vi "http handle content data.vi"(4 "transmit queue":refnum<queue>, 6 "exec queue":refnum<queue>, 9 "server properties":T1={"max url size"=8000, "max header"=8000, "timeout ms"=5000, "max data size"=104857600}, 10 "application request":T2, 11 "TCP Network Connection in":refnum<k5>) -> (3 "abort":bool)   [LabVIEW 2013, in "Basic HTTP server.lvclass"]
uses:
  Basic HTTP server.lvclass
  http request.ctl
  http method.ctl
  URI/url structure.ctl
  HTTP headers/http header data.ctl
  http response.ctl
  http response packet type.ctl
  http server properties.ctl
  http chunked encoding state.ctl
  <vilib>/dlg_ctls.llb/Space Constant.vi
  HTTP headers/http add header to set.vi
  HTTP headers/http headers.lvlib
  URI/uniform resource locator.lvlib
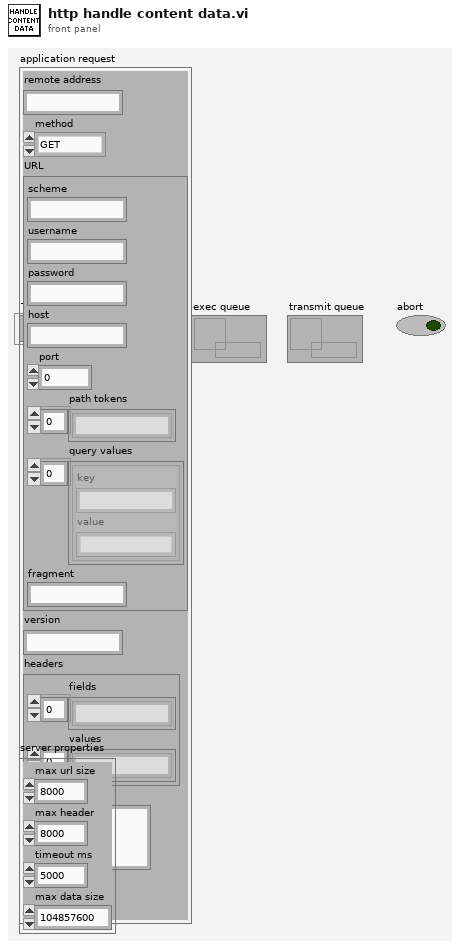
[diagram p1: front panel]
types:
  T1 = typedef "Basic HTTP server.lvclass/http server properties.ctl" = cluster{"max url size":i32, "max header":i32, "timeout ms":i32, "max data size":i32}
  T2 = typedef "Basic HTTP server.lvclass/http request.ctl" = cluster{"remote address":string, "method":T3, "URL":T4, "version":string, "headers":T5, "data":string, "has data?":bool}
  T3 = typedef "Basic HTTP server.lvclass/http method.ctl" = enum16{"GET", "POST", "PUT", "DELETE", "HEAD", "OPTIONS", "upgrade"}
  T4 = typedef "uniform resource locator.lvlib/url structure.ctl" = cluster{"scheme":string, "username":string, "password":string, "host":string, "port":u16, "path tokens":string[], "query values":cluster{"key":string, "value":string}[], "fragment":string}
  T5 = typedef "http headers.lvlib/http header data.ctl" = cluster{"fields":string[], "values":string[]}
  T6 = typedef "Basic HTTP server.lvclass/http chunked encoding state.ctl" = enum16{"length", "data", "trailer"}
  T7 = enum16{"Standard", "Buffered", "CRLF", "Immediate"}
  T8 = typedef "Basic HTTP server.lvclass/http response.ctl" = cluster{"packet type":T9, "reason code":u16, "status string":string, "headers":T5, "cookies":string[], "data":string}
  T9 = typedef "Basic HTTP server.lvclass/http response packet type.ctl" = enum16{"full response", "header only", "data only", "last data"}
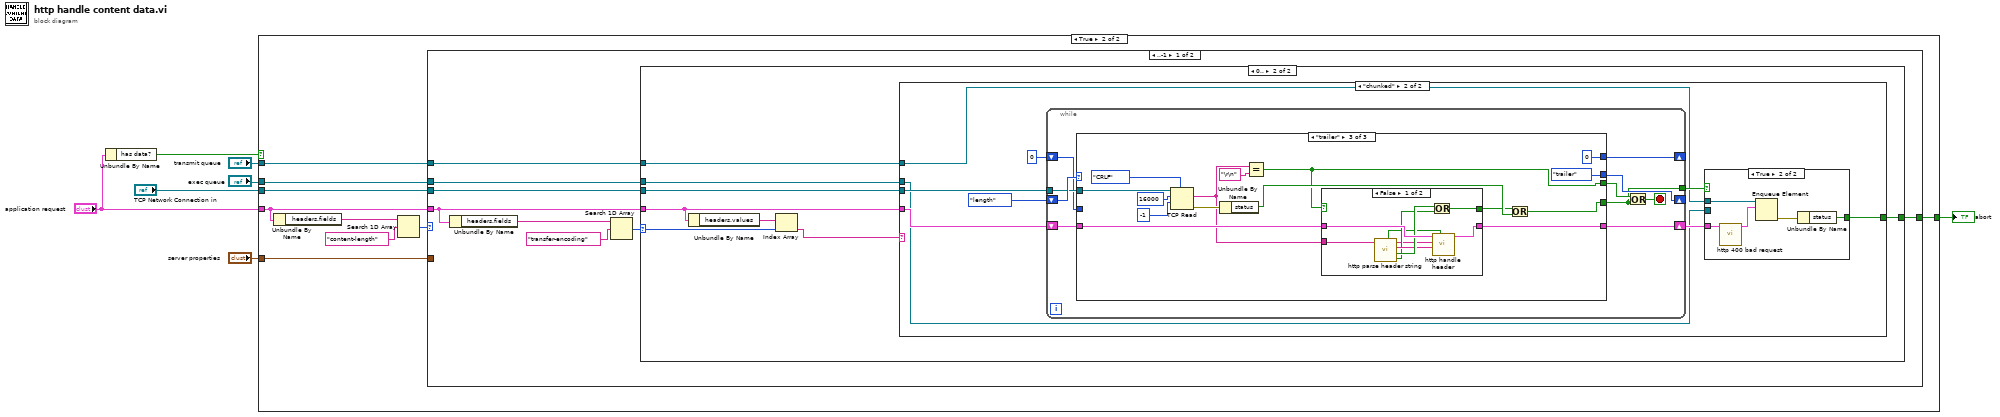
[diagram p0: block diagram]
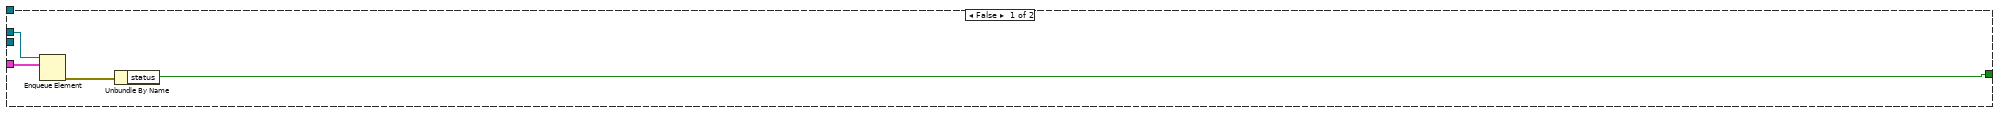
[diagram p2: hidden frame]
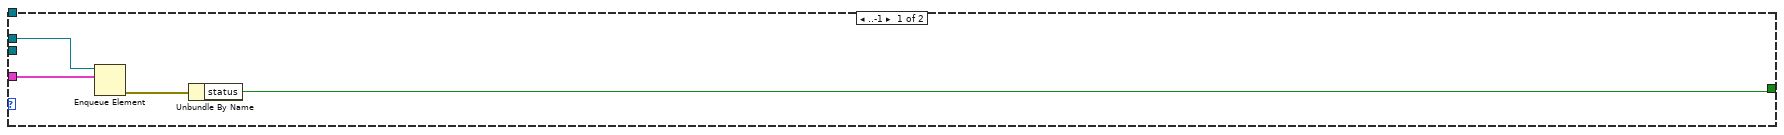
[diagram p3: hidden frame]
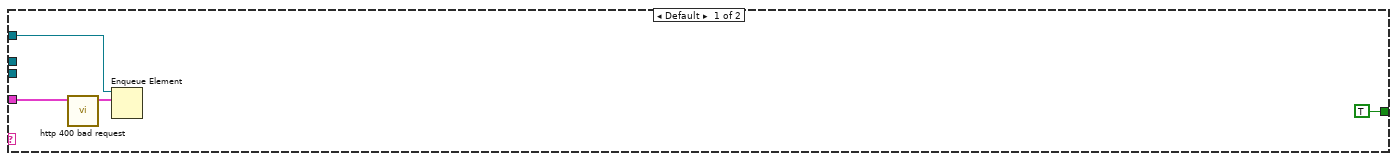
[diagram p4: hidden frame]
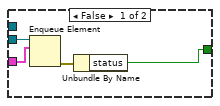
[diagram p5: hidden frame]
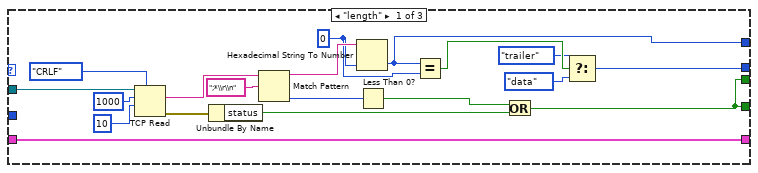
[diagram p6: hidden frame]
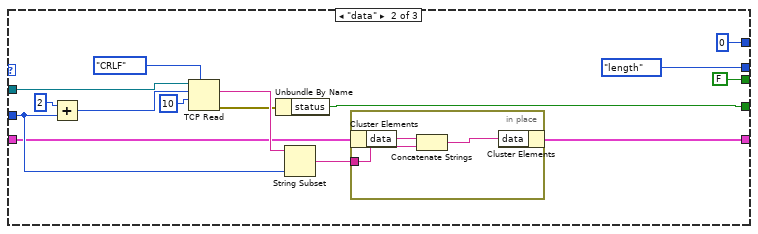
[diagram p7: hidden frame]
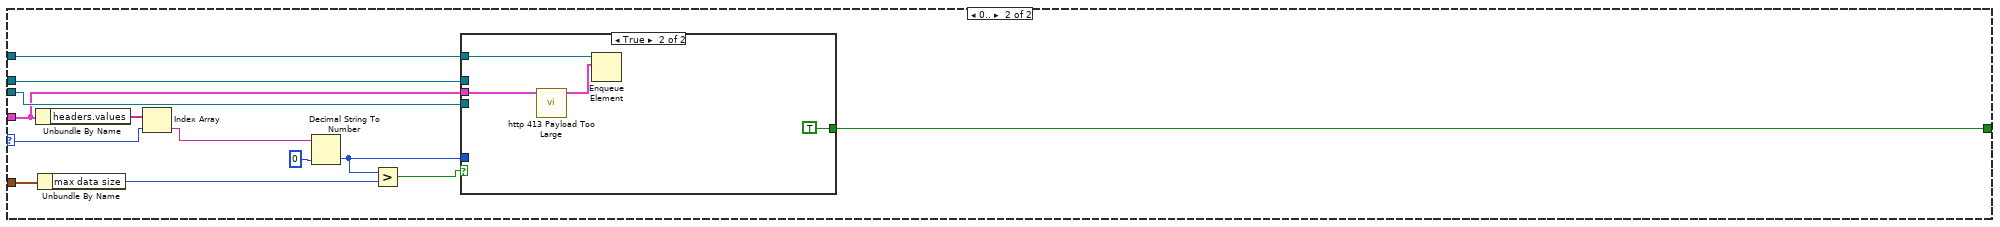
[diagram p9: hidden frame]
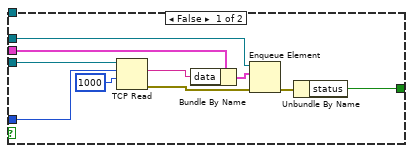
[diagram p10: hidden frame]
diagram:
  n1 = Unbundle By Name("application request") -> ("has data?"=w1:bool)
  n2 = case shown="True" w1 {
    tunnel: "TCP Network Connection in" -> [_ w20]
    tunnel: [w8 w19] -> w6
    tunnel: "server properties" -> [_ w18]
    tunnel: "transmit queue" -> [_ w17]
    tunnel: "exec queue" -> [w10 w16]
    tunnel: "application request" -> [w11 w15]
    frame False {
      n3 = Enqueue Element(queue=w10, element=w11) -> (error out=w9:errorcluster)  [unwired: 2 in, 2 out]
      n4 = Unbundle By Name(w9) -> ("status"=w8:bool)
    }
    frame True {
      n5 = Unbundle By Name(w15) -> ("headers.fields"=w14:string[])
      n6 = Search 1D Array(1D array=w14, element="content-length" ("name")) -> (index of element=w12:i32)  [unwired: 1 in]
      n7 = case shown="..-1" w12 {
        selector: w12 -> [_ w136]
        tunnel: w15 -> [w27 w138]
        tunnel: w20 -> [w26 w146]
        tunnel: [w28 w145] -> w19
        tunnel: w18 -> [_ w144]
        tunnel: w17 -> [w24 w140]
        tunnel: w16 -> [w25 w139]
        frame ..-1 {
          n8 = Unbundle By Name(w27) -> ("headers.fields"=w22:string[])
          n9 = Search 1D Array(1D array=w22, element="transfer-encoding" ("name")) -> (index of element=w21:i32)  [unwired: 1 in]
          n10 = case shown="0.." w21 {
            selector: w21 -> [_ w34]
            tunnel: [w29 w40] -> w28
            tunnel: w27 -> [w32 w36]
            tunnel: w26 -> [_ w39]
            tunnel: w25 -> [w31 w38]
            tunnel: w24 -> [_ w37]
            frame ..-1 {
              n11 = Enqueue Element(queue=w31, element=w32) -> (error out=w30:errorcluster)  [unwired: 2 in, 2 out]
              n12 = Unbundle By Name(w30) -> ("status"=w29:bool)
            }
            frame 0.. {
              n13 = Unbundle By Name(w36) -> ("headers.values"=w35:string[])
              n14 = Index Array(array=w35, index=w34) -> (element=w33:string)
              n15 = case shown="\"chunked\"" w33 {
                tunnel: [TRUE w46] -> w40
                tunnel: w36 -> [w41 w50]
                tunnel: w39 -> [_ w52]
                tunnel: w38 -> [_ w47]
                tunnel: w37 -> [w42 w45]
                frame Default {
                  n16 = call "http 400 bad request.vi"("application request in"=w41) -> ("application request out"=w43:T8)  [unwired: 10 in]
                  n17 = Enqueue Element(queue=w42, element=w43) -> ()  [unwired: 2 in, 3 out]
                }
                frame "chunked" {
                  n18 = while {
                    shift-right: [w70] -> _
                    shift-left: http_chunked_encoding_state."length" -> [w72]
                    tunnel: w52 -> [w71]
                    shift-right: [w68] -> _
                    shift-left: 0 ("default (0 I32)") -> [w67]
                    shift-right: [w65] -> w48
                    shift-left: w50 -> [w66]
                    tunnel: [w63] -> w49
                    stop <- w64 stop-if-true
                    n19 = case shown="\"trailer\"" w72 {
                      tunnel: w71 -> [w91 w104 w121]
                      tunnel: [w78 http_chunked_encoding_state."length" http_chunked_encoding_state."trailer"] -> w70
                      tunnel: [w74 FALSE w115] -> w69
                      tunnel: [w83 0 0] -> w68
                      tunnel: w67 -> [_ w100 _]
                      tunnel: w66 -> [w77 w93 w113]
                      tunnel: [w77 w92 w114] -> w65
                      tunnel: [w74 w94 w112] -> w63
                      frame "length" {
                        w84 = 0 ("default (0 I32)")
                        n20 = TCP Read(connection ID=w91, bytes to read=1000, 7:T7."CRLF" ("mode (standard)"), 9:10 ("timeout ms (25000)")) -> (data out=w87:string, error out=w75:errorcluster)  [unwired: 1 in, 1 out]
                        n21 = Unbundle By Name(w75) -> ("status"=w73:bool)
                        n22 = Match Pattern(string=w87, regular expression=";*\\r\\n") -> (before substring=w85:string, offset past match=w82:i32)  [unwired: 1 in, 2 out]
                        n23 = Hexadecimal String To Number(string=w85, default (0uL)=w84) -> (number=w83:i32)  [unwired: 1 in, 1 out]
                        n24 = Less Than 0?(x=w82) -> (x < 0?=w76:bool)
                        n25 = Equal?(x=w83, y=w84) -> (x = y?=w81:bool)
                        n26 = Or(x=w76, y=w73) -> (x .or. y?=w74:bool)
                        n27 = Select(t=http_chunked_encoding_state."trailer", s=w81, f=http_chunked_encoding_state."data") -> (s? t:f=w78:T6)
                      }
                      frame "data" {
                        n28 = Add(x=2, y=w100) -> (x+y=w103:i32)
                        n29 = TCP Read(connection ID=w104, bytes to read=w103, 7:T7."CRLF" ("mode (standard)"), 9:10 ("timeout ms (25000)")) -> (data out=w101:string, error out=w95:errorcluster)  [unwired: 1 in, 1 out]
                        n30 = Unbundle By Name(w95) -> ("status"=w94:bool)
                        n31 = String Subset(string=w101, length (rest)=w100) -> (substring=w99:string)  [unwired: 1 in]
                        n32 = in-place {
                          in-place-border: w99 -> [w109]
                          n33 = in-place-cluster #1(w93) -> ("data"=w108:string)
                          n34 = Concatenate Strings(w108, w109) -> (w107:string)
                          n35 = in-place-cluster #1("data"=w107) -> (w92:T2)
                        }
                      }
                      frame "trailer" {
                        n36 = TCP Read(connection ID=w121, bytes to read=16000, 7:T7."CRLF" ("mode (standard)"), 9:-1 ("timeout ms (25000)")) -> (data out=w110:string, error out=w119:errorcluster)  [unwired: 1 in, 1 out]
                        n37 = Unbundle By Name(w119) -> ("status"=w118:bool)
                        n38 = Equal?(x=w110, y="\r\n" ("x")) -> (x = y?=w115:bool)
                        n39 = case shown="False" w115 {
                          tunnel: [w133 w134] -> w114
                          tunnel: w113 -> [w132 w134]
                          tunnel: [w128 _] -> w111
                          tunnel: w110 -> [w129 _]
                          frame False {
                            n40 = call "http parse header string.vi"("raw string"=w129) -> ("no field name"=w127:bool, "no crlf"=w131:bool, "header field data"=w130:string, "header field name"=w126:string, "continuation"=w125:bool)  [unwired: 6 in]
                            n41 = Or(x=w131, y=w127) -> (x .or. y?=w128:bool)
                            n42 = call "http handle header.vi"("continuation"=w125, "header field data"=w130, "header field name"=w126, "application request in"=w132) -> ("application request out"=w133:T2)  [unwired: 7 in]
                          }
                          frame True {
                          }
                        }
                        n43 = Or(x=w111, y=w118) -> (x .or. y?=w112:bool)
                      }
                    }
                    n44 = Or(x=w69, y=w63) -> (x .or. y?=w64:bool)
                  }
                  n45 = case shown="True" w49 {
                    tunnel: w48 -> [w56 w60]
                    tunnel: w47 -> [w57 _]
                    tunnel: [w54 w61] -> w46
                    tunnel: w45 -> [_ w58]
                    frame False {
                      n46 = Enqueue Element(queue=w57, element=w56) -> (error out=w55:errorcluster)  [unwired: 2 in, 2 out]
                      n47 = Unbundle By Name(w55) -> ("status"=w54:bool)
                    }
                    frame True {
                      n48 = call "http 400 bad request.vi"("application request in"=w60) -> ("application request out"=w59:T8)  [unwired: 10 in]
                      n49 = Enqueue Element(queue=w58, element=w59) -> (error out=w62:errorcluster)  [unwired: 2 in, 2 out]
                      n50 = Unbundle By Name(w62) -> ("status"=w61:bool)
                    }
                  }
                }
              }
            }
          }
        }
        frame 0.. {
          n51 = Unbundle By Name(w138) -> ("headers.values"=w137:string[])
          n52 = Unbundle By Name(w144) -> ("max data size"=w143:i32)
          n53 = Index Array(array=w137, index=w136) -> (element=w135:string)
          n54 = Decimal String To Number(string=w135, default (0L)=0 ("default (0 I32)")) -> (number=w142:i32)  [unwired: 1 in, 1 out]
          n55 = Greater?(x=w142, y=w143) -> (0:w141:bool)
          n56 = case shown="True" w141 {
            tunnel: w146 -> [w157 _]
            tunnel: [w155 TRUE ("status")] -> w145
            tunnel: w138 -> [w154 w160]
            tunnel: w142 -> [w151 _]
            tunnel: w140 -> [_ w158]
            tunnel: w139 -> [w149 _]
            frame False {
              n57 = TCP Read(connection ID=w157, bytes to read=w151, 9:1000 ("timeout ms (25000)")) -> (data out=w153:string, error out=w152:errorcluster)  [unwired: 2 in, 1 out]
              n58 = Bundle By Name(cluster=w154, "data"=w153) -> (w148:T2)
              n59 = Enqueue Element(queue=w149, element=w148, error in (no error)=w152) -> (error out=w150:errorcluster)  [unwired: 1 in, 2 out]
              n60 = Unbundle By Name(w150) -> ("status"=w155:bool)
            }
            frame True {
              n61 = call "http 413 Payload Too Large.vi"("application request in"=w160) -> ("application request out"=w159:T8)  [unwired: 10 in]
              n62 = Enqueue Element(queue=w158, element=w159) -> ()  [unwired: 2 in, 3 out]
            }
          }
        }
      }
    }
  }
  "abort" <- w6
